vi "Emballage_BDD_bdd_config_emballage.vi"(8 "Error in":errorcluster caption="Error in (no error)", 9 "progress":refnum<vi>, 10 "Refnum Ch":refnum<vi>, 11 "tableau_config":string[][](array[string])) -> (0 "Error out":errorcluster, 3 "db file out":path)   [LabVIEW 2020]
uses:
  Modules/FS/60_FS_Controles/60_FS_SetGet.ctl
  <vilib>/drjdpowell/SQLite Library/SQL Connection/Open (path).vi
  <vilib>/drjdpowell/SQLite Library/SQL Connection/Open (string).vi
  <vilib>/AdvancedString/Path To Command Line String.vi
  <vilib>/drjdpowell/SQLite Library/SQL Connection/Connection.lvclass
panel:
  out "deltaTime [ms]":u32
  out "requete":string
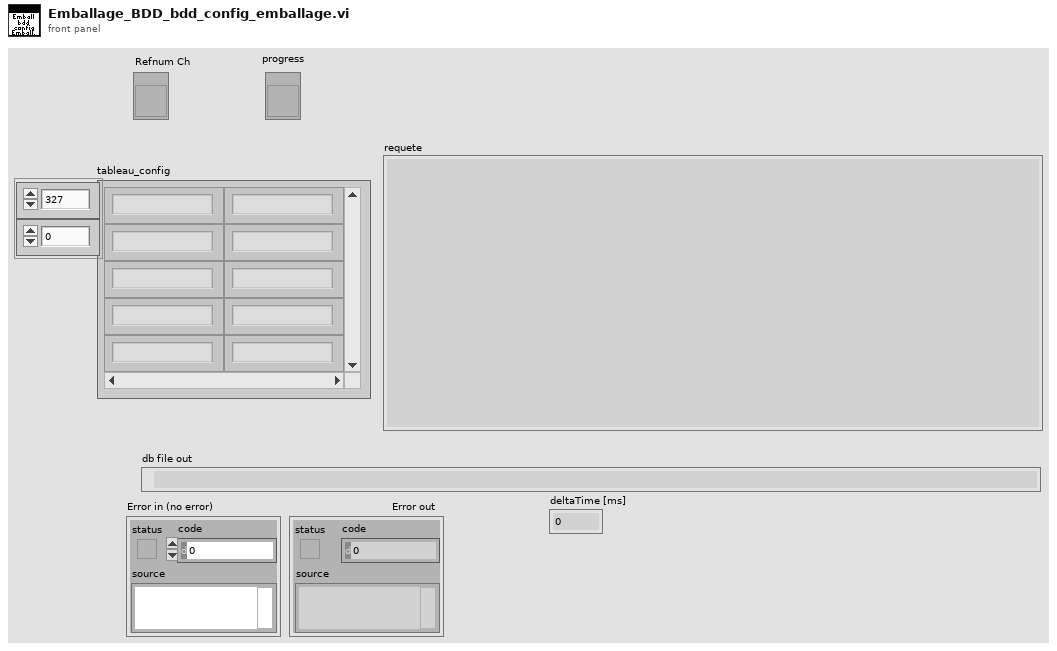
[diagram p1: front panel]
types:
  T1 = typedef "60_FS_SetGet.ctl" = enum16{"set", "get"}
  T2 = typedef "60_FS_CLT_Chemins.ctl" = cluster{"Racine_local":path, "Racine_reseau":path, "Racine_Support_Application":path, "Fichier_Journalisation":path, "Connexion_BDD_VSX":path, "Connexion_BDD_PLZ":path}
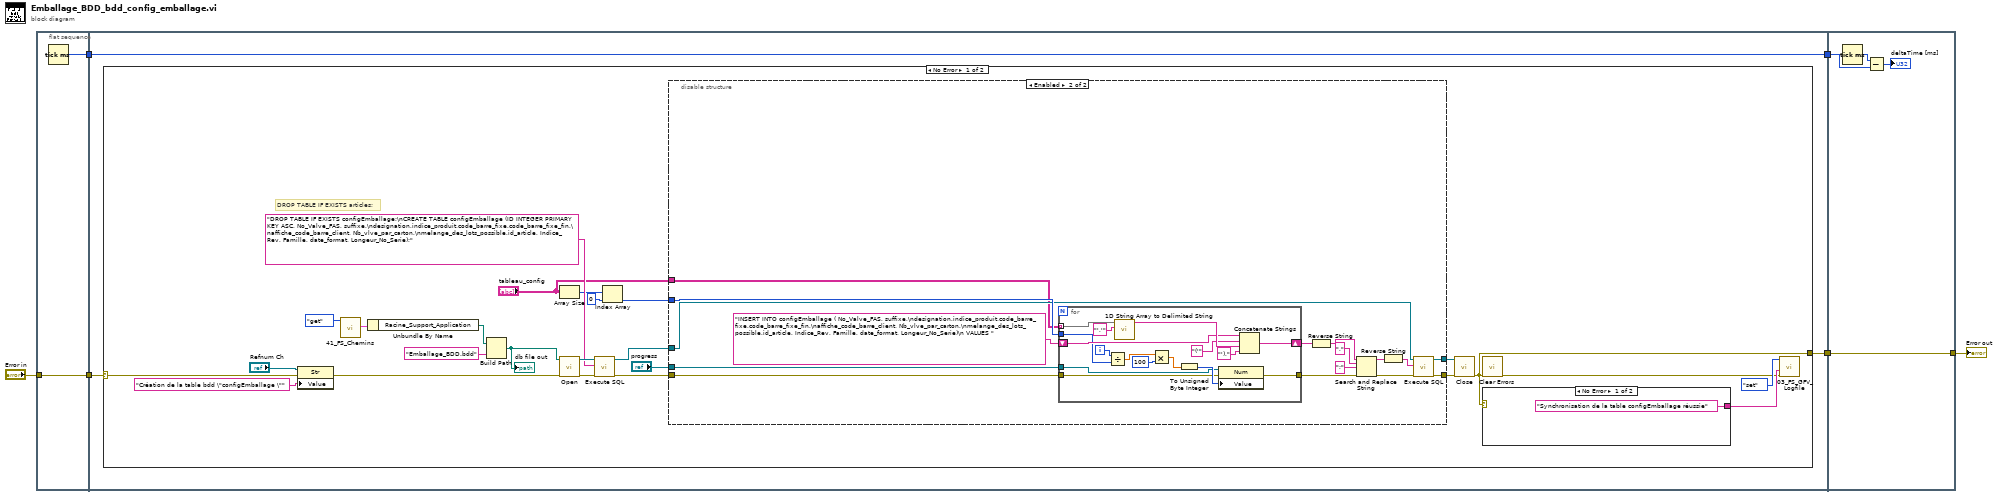
[diagram p0: block diagram]
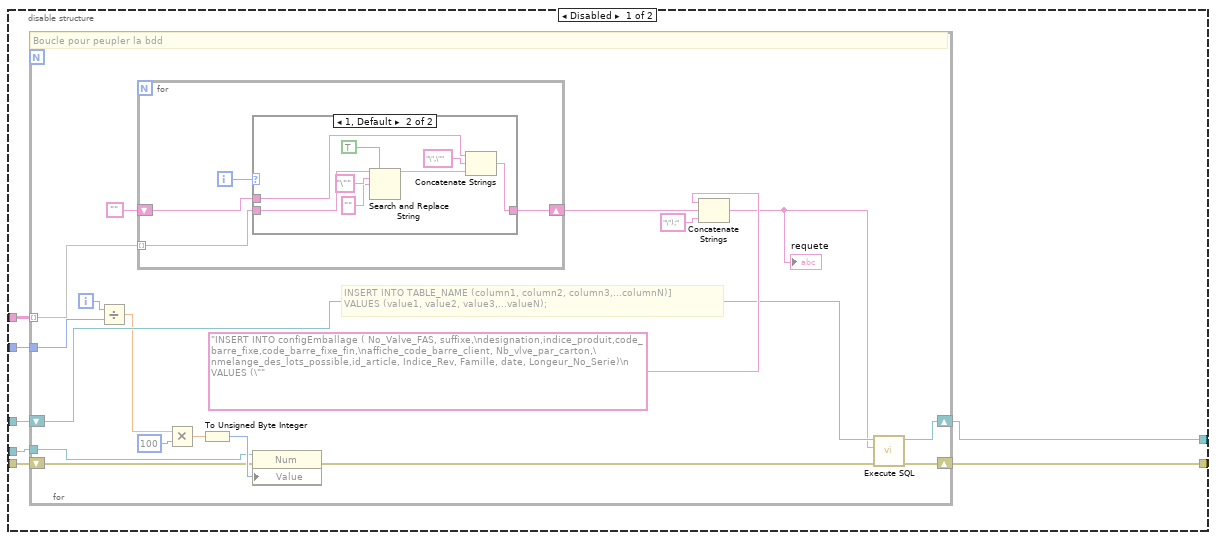
[diagram p2: hidden frame]
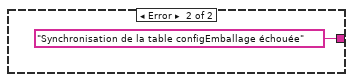
[diagram p4: hidden frame]
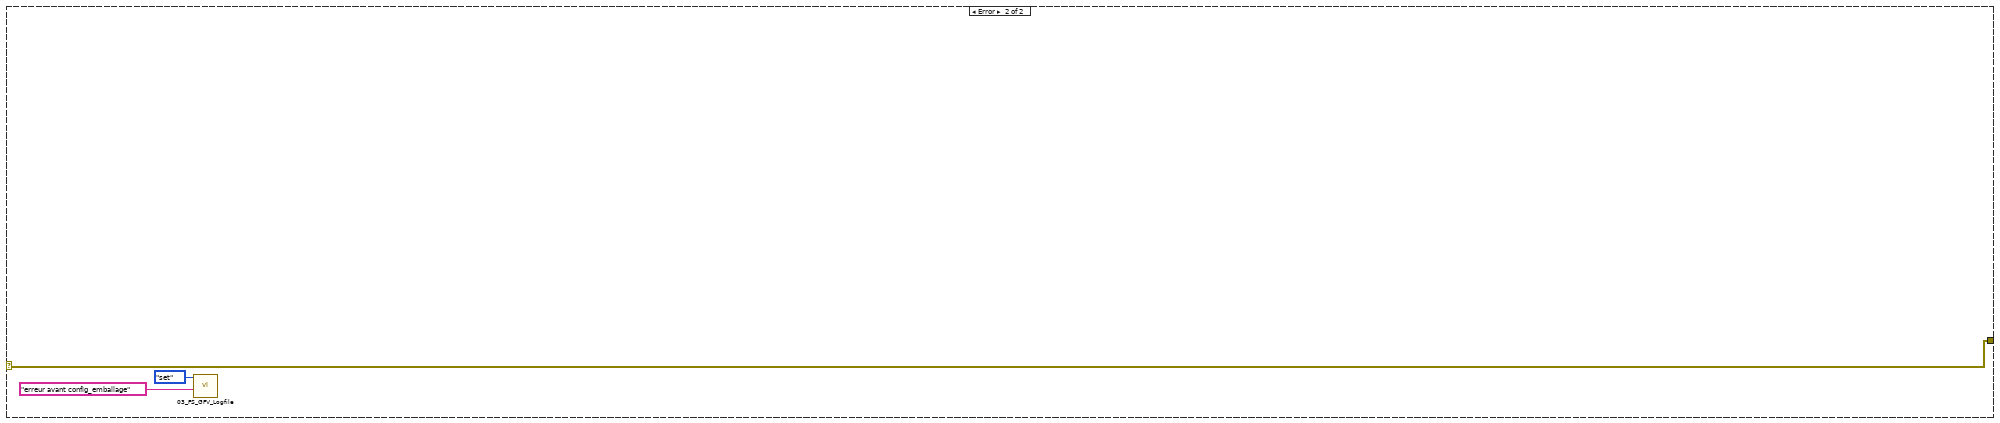
[diagram p5: hidden frame]
diagram:
  n1 = flat-sequence {
    tunnel: "Error in" -> [w8]
    tunnel: [w8] -> w3
    tunnel: [w7] -> w2
    tunnel: [w10] -> w4
    tunnel: w3 -> [w11]
    tunnel: w2 -> [w9]
    tunnel: [w9] -> w1
    tunnel: [w115] -> w5
    tunnel: w4 -> [w115]
    tunnel: w1 -> [w113]
    frame #0 {
      n2 = Tick Count (ms)() -> (millisecond timer value=w7:u32)
    }
    frame #1 {
      n3 = case shown="No Error" w11 {
        selector: w11 -> [w20 w111]
        tunnel: [w12 w111] -> w10
        frame No Error {
          # "DROP TABLE IF EXISTS articles;"
          n4 = property class="Str"(reference="Refnum Ch", error in=w20, "Value"="Création de la table bdd \"configEmballage \"" ("Valeur")) -> (error out=w19:errorcluster)  [unwired: 1 out]
          n5 = call "41_FS_Chemins.vi"("SetGet"=60_FS_SetGet."get") -> ("CLT_Chemins_out"=w25:T2)  [unwired: 9 in, 1 out]
          n6 = Unbundle By Name(w25) -> ("Racine_Support_Application"=w24:path)
          n7 = Build Path(base path=w24, name or relative path="Emballage_BDD.bdd" ("nom ou chemin relatif")) -> (appended path=w23:path)
          "db file out" <- w23
          n8 = Array Size(array="tableau_config") -> (size(s)=w15:i32[])
          n9 = call-poly <vilib>:"Open.vi"("error in (no error)"=w19, "db file"=w23) -> ("error out"=w35:errorcluster, "SQLite Connection"=w36:refnum<class "Connection.lvclass">)  [unwired: 8 in]
          n10 = call <vilib>:"Execute SQL.vi"("error in (no error)"=w35, "SQL"="DROP TABLE IF EXISTS configEmballage;\nCREATE TABLE configEmballage (ID INTEGER PRIMARY KEY ASC, No_Valve_FAS, suffixe,\ndesignation,indice_produit,code_barre_fixe,code_barre_fixe_fin,\naffiche_code_barre_client, Nb_vlve_par_carton,\nmelange_des_lots_possible,id_article, Indice_Rev, Famille, date_format, Longeur_No_Serie);", "SQLite Connection in"=w36) -> ("error out"=w33:errorcluster, "SQLite Connection"=w31:refnum<class "Connection.lvclass">)  [unwired: 5 in, 2 out]
          n11 = Index Array(array=w15, index=0 ("indice")) -> (element=w13:i32)
          n12 = disable-structure shown="Enabled" {
            disable-tunnel: w33 -> [w43 w80]
            disable-tunnel: [w42 w78] -> w32
            disable-tunnel: w31 -> [w41 w76]
            disable-tunnel: [w40 w77] -> w30
            disable-tunnel: "progress" -> [w39 w82]
            disable-tunnel: "tableau_config" -> [w38 w75]
            disable-tunnel: w13 -> [w37 w81]
            frame Disabled {
              n13 = for {
                tunnel: w38 -> [w61] mode=indexing
                shift-right: [w55] -> w40
                shift-left: w41 -> [w56]
                shift-right: [w57] -> w42
                shift-left: w43 -> [w47]
                tunnel: w39 -> [w45]
                tunnel: w37 -> [w44]
                i -> [w49]
                # "INSERT INTO TABLE_NAME (column1, column2, column3,...columnN)]  \nVALUES (value1, value2, value3,...valueN);"
                # "Boucle pour peupler la bdd"
                n14 = Divide(x=w49, y=w44) -> (x/y=w52:dbl)
                n15 = for {
                  shift-right: [w65] -> w58
                  shift-left: "" -> [w64]
                  tunnel: w61 -> [w62] mode=indexing
                  i -> [w63]
                  n16 = case shown="1, Default" w63 {
                    tunnel: [w66 w74] -> w65
                    tunnel: w64 -> [_ w73]
                    tunnel: w62 -> [w66 w70]
                    frame 0 {
                    }
                    frame 1, Default {
                      n17 = Search and Replace String(replace all?=TRUE ("tout remplacer ? (F)"), input string=w70, search string="\"" ("chaîne recherchée"), replace string="" ("chaîne de remplacement (\"\")")) -> (result string=w71:string)  [unwired: 4 in, 3 out]
                      n18 = Concatenate Strings(w73, "\",\"" ("chaîne"), w71) -> (w74:string)
                    }
                  }
                }
                n19 = Multiply(x=w52, y=u8 100) -> (x*y=w50:dbl)
                n20 = To Unsigned Byte Integer(number=w50) -> (unsigned 8bit integer=w48:u8)
                n21 = property class="Num"(reference=w45, error in=w47, "Value"=w48) -> (error out=w46:errorcluster)  [unwired: 1 out]
                n22 = Concatenate Strings("INSERT INTO configEmballage ( No_Valve_FAS, suffixe,\ndesignation,indice_produit,code_barre_fixe,code_barre_fixe_fin,\naffiche_code_barre_client, Nb_vlve_par_carton,\nmelange_des_lots_possible,id_article, Indice_Rev, Famille, date, Longeur_No_Serie)\n VALUES (\"" ("SQL"), w58, "\");" ("chaîne")) -> (w54:string)
                "requete" <- w54
                n23 = call <vilib>:"Execute SQL.vi"("error in (no error)"=w46, "SQL"=w54, "SQLite Connection in"=w56) -> ("error out"=w57:errorcluster, "SQLite Connection"=w55:refnum<class "Connection.lvclass">)  [unwired: 5 in, 2 out]
              }
            }
            frame Enabled {
              n24 = for {
                tunnel: w75 -> [w106] mode=indexing
                shift-right: [w104] -> w86
                shift-left: "INSERT INTO configEmballage ( No_Valve_FAS, suffixe,\ndesignation,indice_produit,code_barre_fixe,code_barre_fixe_fin,\naffiche_code_barre_client, Nb_vlve_par_carton,\nmelange_des_lots_possible,id_article, Indice_Rev, Famille, date_format, Longeur_No_Serie)\n VALUES " ("SQL") -> [w96]
                tunnel: [w95] -> w90
                tunnel: w82 -> [w94]
                tunnel: w81 -> [w93]
                tunnel: w80 -> [w91]
                i -> [w92]
                n25 = Divide(x=w92, y=w93) -> (x/y=w97:dbl)
                n26 = call <vilib>:"1D String Array to Delimited String.vi"("delimiter"="','", "string array"=w106) -> ("delimited string"=w103:string)  [unwired: 9 in]
                n27 = Multiply(x=w97, y=u8 100) -> (x*y=w99:dbl)
                n28 = To Unsigned Byte Integer(number=w99) -> (unsigned 8bit integer=w100:u8)
                n29 = property class="Num"(reference=w94, error in=w91, "Value"=w100) -> (error out=w95:errorcluster)  [unwired: 1 out]
                n30 = Concatenate Strings(w96, "('" ("string"), w103, "')," ("string")) -> (w104:string)
              }
              n31 = Reverse String(1:w86) -> (0:w89:string)
              n32 = Search and Replace String(input string=w89, search string=",", replace string=";" ("replace string (\"\")"), error in=w90) -> (result string=w88:string, error out=w79:errorcluster)  [unwired: 4 in, 2 out]
              n33 = Reverse String(1:w88) -> (0:w87:string)
              n34 = call <vilib>:"Execute SQL.vi"("error in (no error)"=w79, "SQL"=w87, "SQLite Connection in"=w76) -> ("error out"=w78:errorcluster, "SQLite Connection"=w77:refnum<class "Connection.lvclass">)  [unwired: 5 in, 2 out]
            }
          }
          n35 = call-dynamic "Close.vi"("error in (no error)"=w32, "SQLite Connection in"=w30) -> ("error out"=w12:errorcluster)  [unwired: 9 in]
          n36 = call <vilib>:"Clear Errors.vi"("error in (no error)"=w12) -> ("error out"=w27:errorcluster)  [unwired: 5 in, 1 out]
          n37 = case shown="No Error" w12 {
            tunnel: ["Synchronisation de la table configEmballage réussie" ("Chaîne") "Synchronisation de la table configEmballage échouée" ("Chaîne")] -> w28
            frame No Error {
            }
            frame Error {
            }
          }
          n38 = call "03_FS_GFV_Logfile.vi"("error in"=w27, "Chaîne"=w28, "States"=60_FS_SetGet."set") -> ()  [unwired: 7 in, 2 out]
        }
        frame Error {
          n39 = call "03_FS_GFV_Logfile.vi"("Chaîne"="erreur avant config_emballage", "States"=60_FS_SetGet."set") -> ()  [unwired: 8 in, 2 out]
        }
      }
    }
    frame #2 {
      n40 = Tick Count (ms)() -> (millisecond timer value=w114:u32)
      n41 = Subtract(x=w114, y=w113) -> (x-y=→"deltaTime [ms]":u32)
    }
  }
  "Error out" <- w5
